vi "Program_EBN_Yann_Berton.vi"() -> ()   [LabVIEW 2020]
uses:
  <instrlib>/Keithley 27XX/Public/Configure/Measurement Specific/Configure Thermocouple.vi
  <instrlib>/Keithley 27XX/Public/Configure/Measurement Specific/Configure FRTD.vi
  <instrlib>/Keithley 27XX/Keithley 27XX.lvlib
panel:
  in  "Number of samples allowed":dbl=15.0
  out "Close 50 mbar valve":bool
  out "T_ts_in_mid (wall)":dbl
  out "T_ts_in_top (wall)":dbl
  out "T_out_ts_mid (wall)":dbl
  out "T_out_ts_bot (wall)":dbl
  out "Counter":dbl
  out "T_PH_surf4":dbl
  out "T_PH_surf3":dbl
  out "TCHF_bot":dbl
  out "TCHF_top":dbl
  out "T3_bot":dbl
  out "T3_mid":dbl
  out "T3_top":dbl
  out "T2_top":dbl
  out "T2_mid":dbl
  out "T2_bot":dbl
  out "T1_top":dbl
  out "T1_mid":dbl
  out "T1_bot":dbl
  out "T_PH_surf2":dbl
  out "Absolute pressure":dynamicdata(graph)
  out "Pressure drop":dynamicdata(graph)
  out "Temperatures":dynamicdata(graph)
  in  "Porta RS232 Keithley 2701":refnum<visa-resource-name>="COM1"
  in  "Aquisition {Sample/s]":u32=1
  in  "stop":bool
  out "stop flag":bool
  out "V_TS_corr2":dbl
  out "P_reservoir (kPa)":dbl
  out "P_TS_in (kPa)":dbl
  out "P_pump_in (kPa)":dbl
  out "mass (kg/s)":dbl
  out "0-50 mbar (kPa)":dbl
  out "0-2 bar (kPa)":dbl
  out "T_ph_in (imm)":dbl
  out "T_amb":dbl
  out "T_reserv_bot":dbl
  out "T_reser_top":dbl
  out "T_TS_out_top (wall)":dbl
  out "T_TS_out (imm)":dbl
  out "T_PH_surf1":dbl
  out "T_PH_in (wall)":dbl
  out "T_TS_in (imm)":dbl
  out "T_TS_in_bot (wall)":dbl
  out "T_pump_in":dbl
  in  "File":path=path "C:/test.lvm" caption="Filename"
  in  "Save":bool caption="Enable"
  out "0-5 bar (kPa)":dbl
  out "Tcj ch201":dbl
  # "SAVING DATA"
  # "Pre-heater temperatures"
  # "Test section temperatures"
  # "85 mm mm"
  # "40 mm"
  # "62.5 mm mm"
  # "665 mm"
  # "1347 mm mm"
  # "115 mm mm"
  # "809 mm"
  # "1585 mm mm"
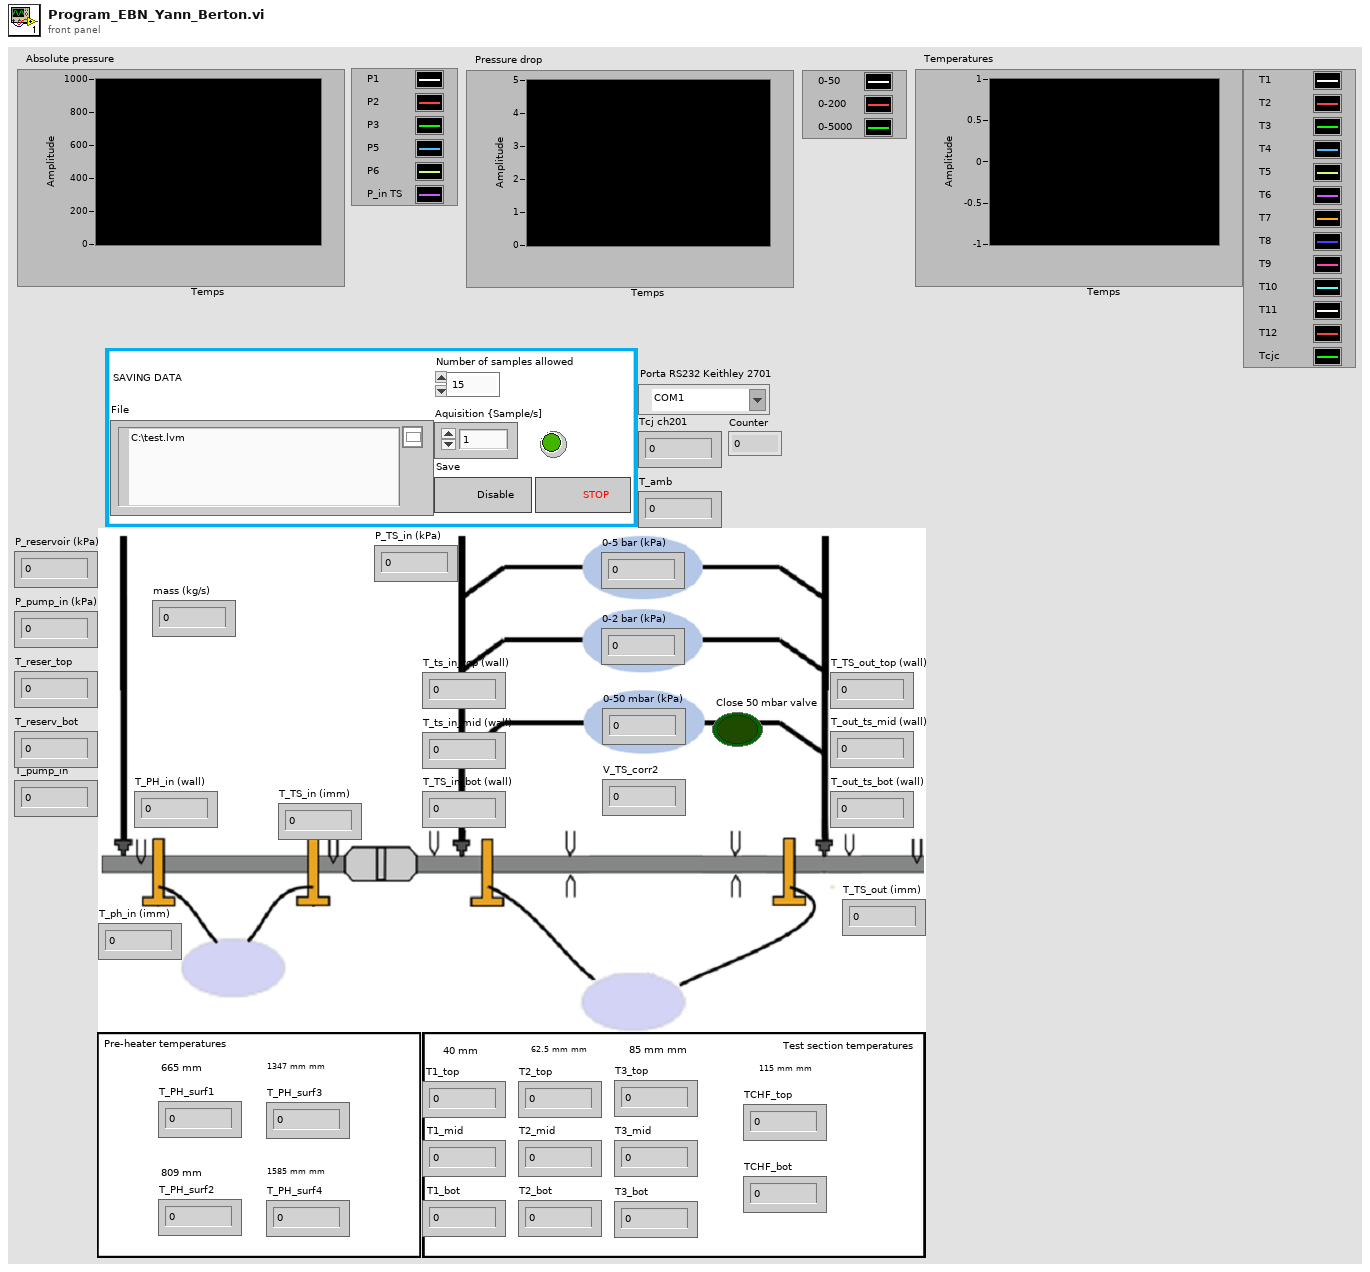
[diagram p1: front panel]
types:
  T1 = cluster{"Baud Rate (9600)":u32, "Flow Control (1: XON/XOFF)":u16, "Termination Char (0:CR)":u16}
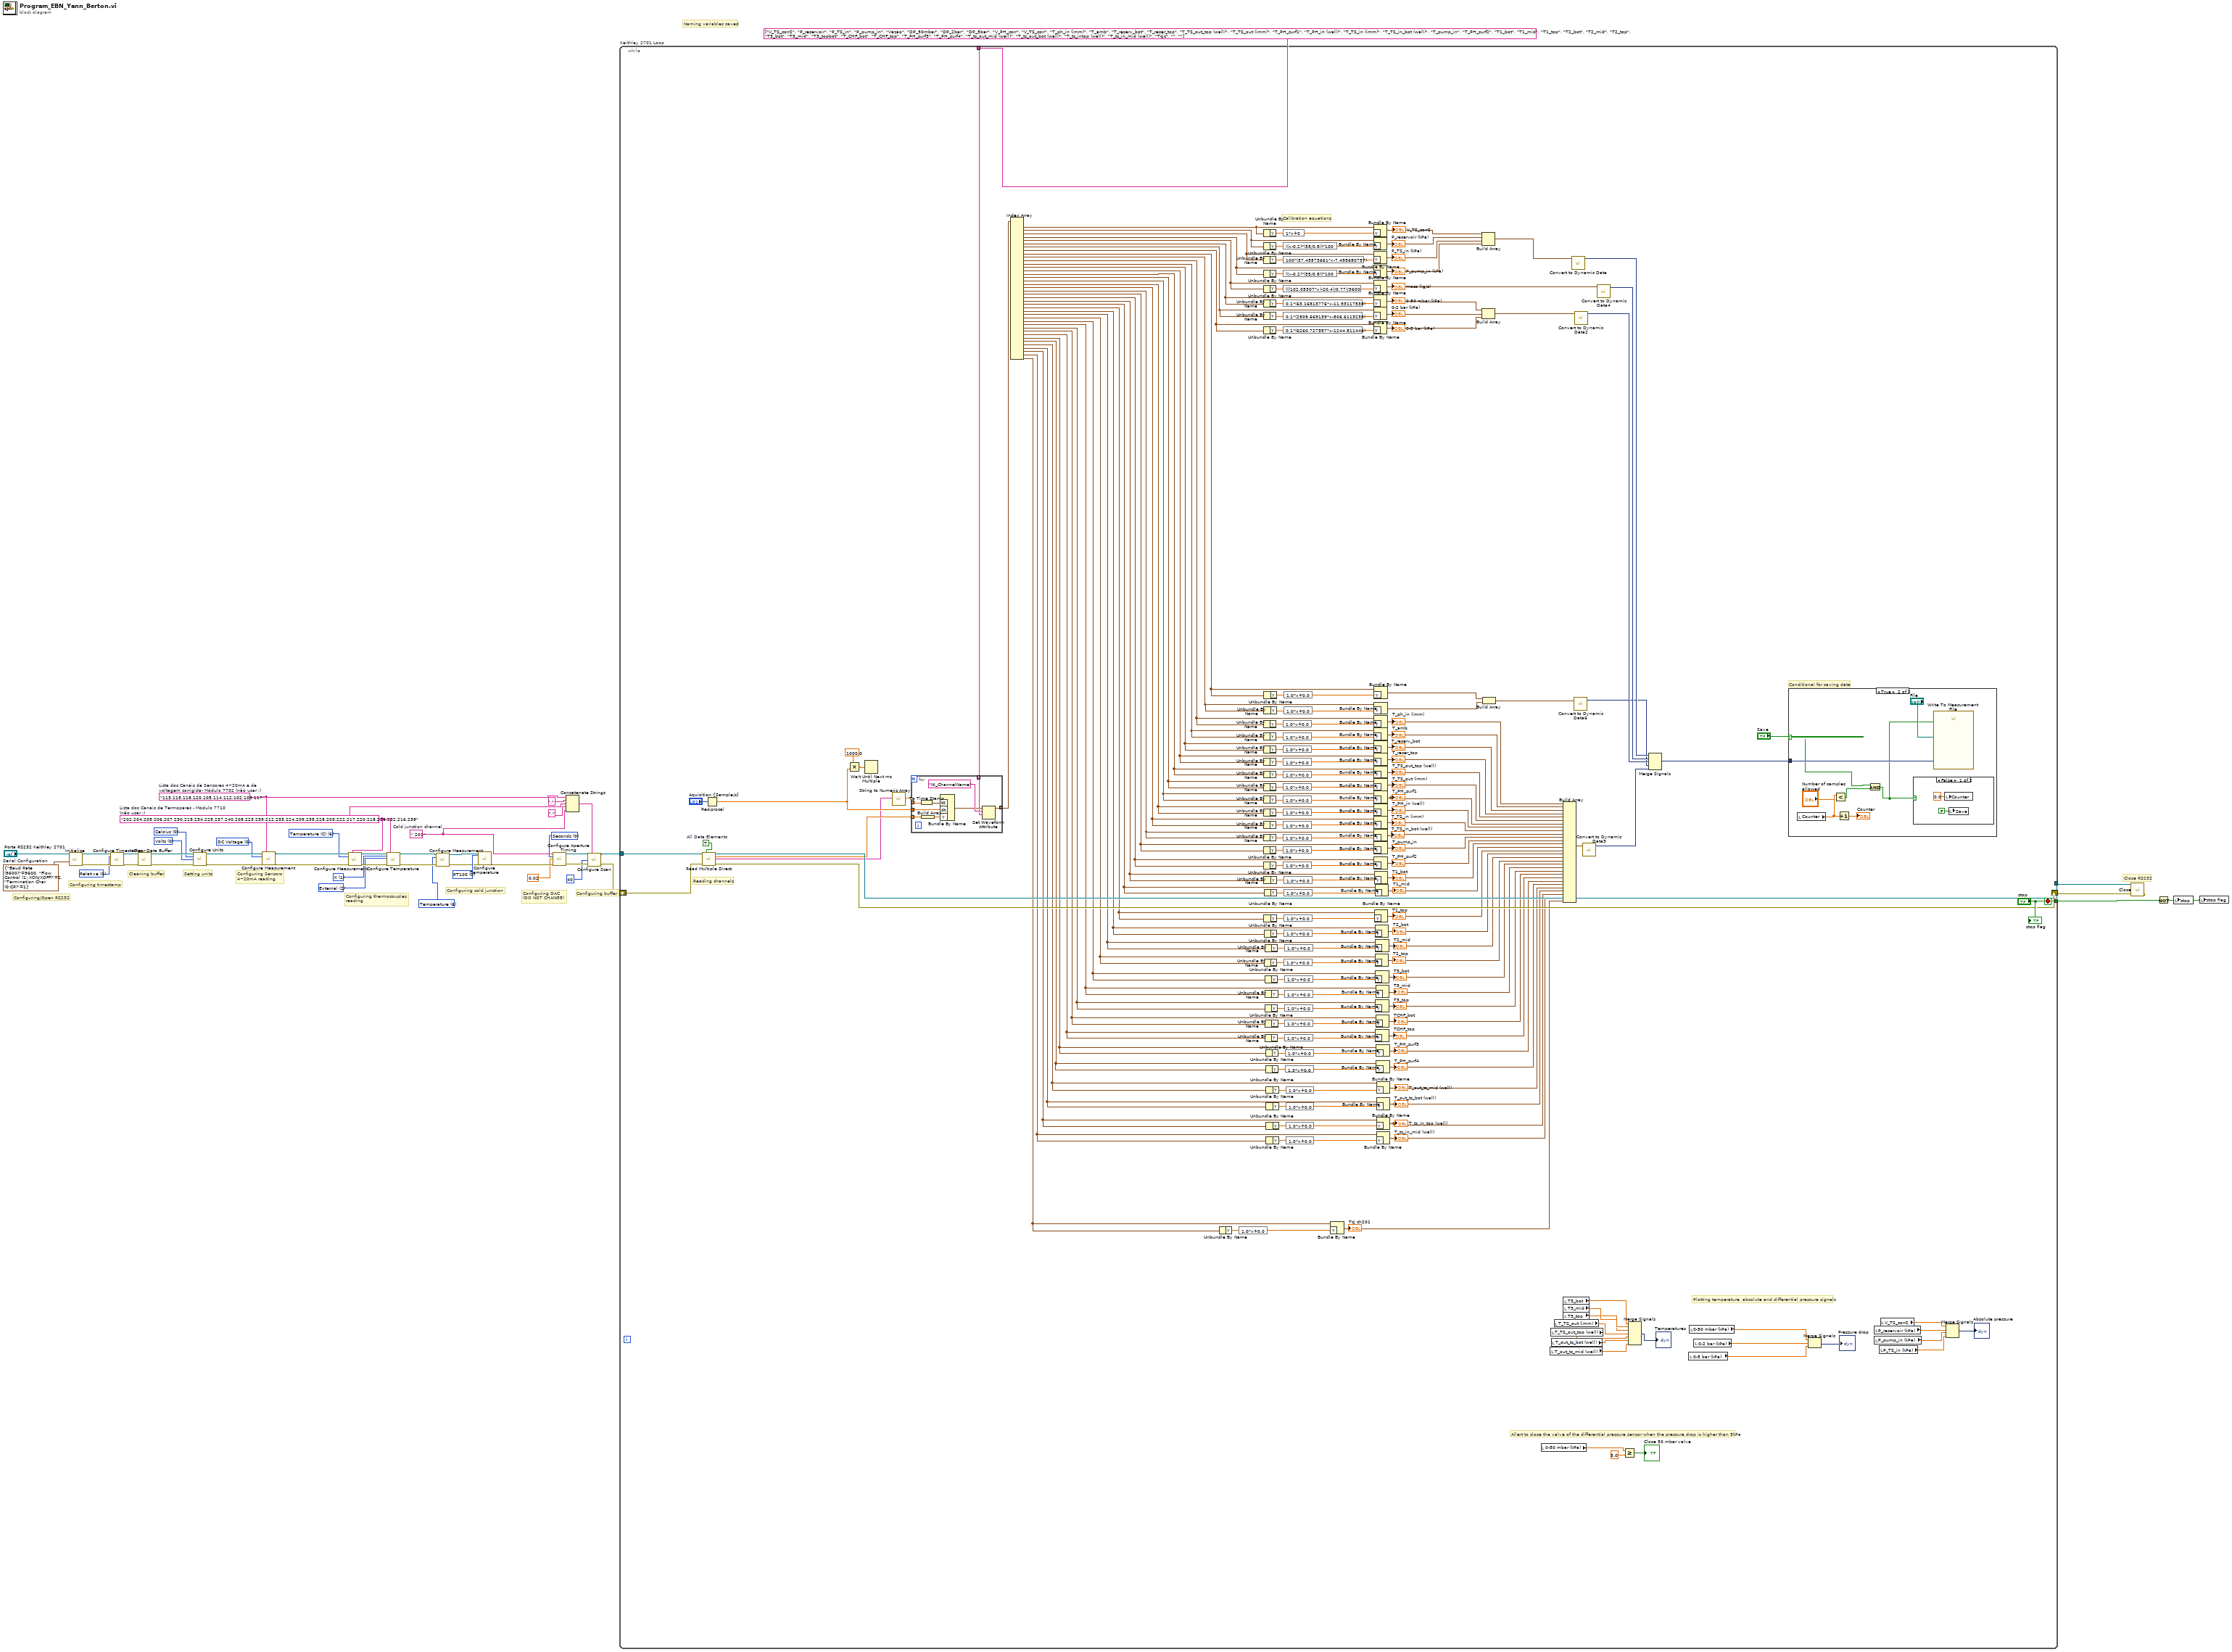
[diagram p0: block diagram]
diagram:
  w15 = u16 0 items=["PT100", "D100", "F100", "PT3916", "PT385", "USER"] ("FRTD Type (0: PT100)")
  w17 = u16 6 items=["DC Voltage", "AC Voltage", "DC Current", "AC Current", "Resistance", "Four-Wire Resistance", "Temperature", "Frequency", "Period", "Continuity"] ("Function (0: DC Voltage)")
  w1 = " 201"  # Cold junction channel
  w23 = "202,204,205,206,207,230,219,234,225,237,240,208,223,239,212,233,224,209,235,228,203,222,217,220,218,226,232,216,238"  # Lista dos Canais de Termopares - Módulo 7710 (não usar :)
  w31 = "113,115,118,120,105,114,112,102,109,117"  # Lista dos Canais de Sensores 4~20mA e de voltagem corrigida- Módulo 7702 (não usar :)
  w12 = u16 0 items=["Seconds", "Power Line Cycles"] ("Timing Units (0: Seconds)")
  w20 = u16 2 items=["Simulated", "Internal", "External"] ("Reference Junction Type (0: Simulated)")
  w21 = u16 1 items=["J", "K", "T", "E", "R", "S", "B", "N"] ("Thermocouple Type (1: K)")
  w32 = u16 0 items=["Volts", "dB"] ("DC Voltage (0: V)")
  w33 = u16 0 items=["Celsius", "Fahrenheit", "Kelvin"] ("Temperature (0: Celsius)")
  w25 = u16 6 items=["DC Voltage", "AC Voltage", "DC Current", "AC Current", "Resistance", "Four-Wire Resistance", "Temperature (C)", "Frequency", "Period", "Continuity"] ("Function (0: DC Voltage)")
  w28 = u16 0 items=["DC Voltage", "AC Voltage", "DC Current", "AC Current", "Resistance", "Four-Wire Resistance", "Temperature (C)", "Frequency", "Period", "Continuity"] ("Function (0: DC Voltage)")
  w41 = T1 {"Baud Rate (9600)"=9600, "Flow Control (1: XON/XOFF)"=2, "Termination Char (0:CR)"=1}  # Serial Configuration
  w38 = u16 0 items=["Relative", "Real Time Clock"] ("Timestamp Type (0: Relative)")
  # "Configuring cold junction"
  # "Naming variables saved"
  # "Close RS232"
  # "Configuring buffer"
  # "Configuring DAC \n(DO NOT CHANGE)"
  # "Configuring thermocouples\nreading"
  # "Configuring Sensors \n4~20mA reading"
  # "Setting units"
  # "Cleaning buffer"
  # "Configuring timestamp"
  # "Configuring/Open RS232"
  n1 = call <instrlib>:"Initialize.vi"("VISA resource name"="Porta RS232 Keithley 2701", "Serial Configuration"=w41) -> ("VISA resource name out"=w40:refnum<visa-resource-name>, "error out"=w39:errorcluster)  [unwired: 12 in]
  n2 = call <instrlib>:"Configure Timestamp.vi"("VISA resource name"=w40, "Timestamp Type (0: Relative)"=w38, "error in (no error)"=w39) -> ("VISA resource name out"=w37:refnum<visa-resource-name>, "error out"=w36:errorcluster)  [unwired: 11 in]
  n3 = call <instrlib>:"Clear Data Buffer.vi"("VISA resource name"=w37, "error in (no error)"=w36) -> ("VISA resource name out"=w35:refnum<visa-resource-name>, "error out"=w34:errorcluster)  [unwired: 12 in]
  n4 = call <instrlib>:"Configure Units.vi"("VISA resource name"=w35, "Temperature (0: Celsius)"=w33, "DC Voltage (0: V)"=w32, "error in (no error)"=w34) -> ("VISA resource name out"=w29:refnum<visa-resource-name>, "error out"=w30:errorcluster)  [unwired: 10 in]
  n5 = call <instrlib>:"Configure Measurement.vi"("VISA resource name"=w29, "Scan List (Empty)"=w31, "Function (0: DC Voltage)"=w28, "error in (no error)"=w30) -> ("VISA resource name out"=w27:refnum<visa-resource-name>, "error out"=w26:errorcluster)  [unwired: 10 in]
  n6 = call <instrlib>:"Configure Measurement.vi"("VISA resource name"=w27, "Scan List (Empty)"=w23, "Function (0: DC Voltage)"=w25, "error in (no error)"=w26) -> ("VISA resource name out"=w24:refnum<visa-resource-name>, "error out"=w22:errorcluster)  [unwired: 10 in]
  n7 = call-poly <instrlib>:"Configure Temperature.vi"("VISA resource name"=w24, "Thermocouple Type (1: K)"=w21, "Reference Junction Type (0: Simulated)"=w20, "error in (no error)"=w22, "Scan List (Empty)"=w23) -> ("VISA resource name out"=w19:refnum<visa-resource-name>, "error out"=w18:errorcluster)  [unwired: 13 in]
  n8 = call <instrlib>:"Configure Measurement.vi"("VISA resource name"=w19, "Function (0: DC Voltage)"=w17, "error in (no error)"=w18) -> ("VISA resource name out"=w16:refnum<visa-resource-name>, "error out"=w14:errorcluster)  [unwired: 11 in]
  n9 = call-poly <instrlib>:"Configure Temperature.vi"("VISA resource name"=w16, "FRTD Type (0: PT100)"=w15, "error in (no error)"=w14) -> ("error out"=w13:errorcluster)  [unwired: 15 in, 1 out]
  n10 = call <instrlib>:"Configure Aperture Timing.vi"("VISA resource name"=w1, "Timing Units (0: Seconds)"=w12, "Timing Value (0.020)"=0.02, "error in (no error)"=w13) -> ("VISA resource name out"=w9:refnum<visa-resource-name>, "error out"=w8:errorcluster)  [unwired: 10 in]
  n11 = Concatenate Strings(w31, "," ("string"), w23, "," ("string"), w1) -> (w10:string)
  n12 = call <instrlib>:"Configure Scan.vi"("VISA resource name"=w9, "Channel List (101:110)"=w10, "Sample Count (100)"=40 ("Sample Count (10)"), "error in (no error)"=w8) -> ("VISA resource name out"=w6:refnum<visa-resource-name>, "error out"=w7:errorcluster)  [unwired: 10 in]
  n13 = while "Keithley 2701 Loop" {
    tunnel: w6 -> [w197]
    tunnel: [w194] -> w4
    shift-right: [w195] -> w3
    shift-left: w7 -> [w196]
    tunnel: string[] ["V_TS_corr2", "P_reservoir", "P_TS_in", "P_pump_in", "Vazao", "DP_50mbar", "DP_2bar", "DP_5bar", "V_PH_corr", "V_TS_corr", "T_ph_in (imm)", "T_amb", "T_reserv_bot", "T_reser_top", "T_TS_out_top (wall)", "T_TS_out (imm)", "T_PH_surf1", "T_PH_in (wall)", "T_TS_in (imm)", "T_TS_in_bot (wall)", "T_pump_in", "T_PH_surf2", "T1_bot", "T1_mid", "T1_top", "T2_bot", "T2_mid", "T2_top", "T3_bot", "T3_mid", "T3_topbot", "T_CHF_bot", "T_CHF_top", "T_PH_surf3", "T_PH_surf4", "T_ts_out_mid (wall)", "T_ts_out_bot (wall)", "T_ts_intop (wall)", "T_ts_in_mid (wall)", "Tcjc", "", ""] -> [w248]
    tunnel: ["stop"] -> w2
    stop <- "stop" stop-if-true
    w190 = TRUE  # All Data Elements
    # "Allert to close the valve of the differential pressure sensor when the pressure drop is higher than 5kPa"
    # "Plotting temperature, absolute and differential pressure signals"
    # "Conditional for saving data"
    # "Calibration equations"
    # "Reading channels"
    n14 = call <instrlib>:"Read Multiple Direct.vi"("VISA resource name"=w197, "All Data Elements (False)"=w190, "error in (no error)"=w196) -> ("VISA resource name out"=w194:refnum<visa-resource-name>, "Measurement Data"=w193:dbl[], "Time Stamp"=w192:string[], "error out"=w195:errorcluster)  [unwired: 7 in, 2 out]
    n15 = Reciprocal(x="Aquisition {Sample/s]") -> (1/x=w249:dbl)
    n16 = Multiply(x=1000.0 ("y"), y=w249) -> (x*y=w250:dbl)
    n17 = Wait Until Next ms Multiple(millisecond multiple=w250) -> ()  [unwired: 1 out]
    n18 = call <instrlib>:"String to Numeric Array.vi"("String Array"=w192) -> ("Numeric Array"=w191:dbl[])  [unwired: 10 in]
    n19 = for {
      tunnel: w191 -> [w271] mode=indexing
      tunnel: w193 -> [w269] mode=indexing
      tunnel: w249 -> [w267]
      tunnel: w248 -> [w264] mode=indexing
      tunnel: [w263] -> w247 mode=indexing
      n20 = To Time Stamp(1:w271) -> (0:w270:timestamp)
      n21 = Build Array(w269) -> (w268:dbl[])
      n22 = Bundle By Name("t0"=w270, "dt"=w267, "Y"=w268) -> (w265:waveform(dbl))  [unwired: 1 in]
      n23 = Set Waveform Attribute(5:w264, 6:"NI_ChannelName" ("name"), 7:w265) -> (3:w263:waveform(dbl))  [unwired: 1 in, 2 out]
    }
    n24 = Index Array(array=w247) -> (element #1=w161:waveform(dbl), element #2=w160:waveform(dbl), element #3=w159:waveform(dbl), element #4=w158:waveform(dbl), element #5=w157:waveform(dbl), element #6=w156:waveform(dbl), element #7=w54:waveform(dbl), element #8=w155:waveform(dbl), element #9=w148:waveform(dbl), element #10=w145:waveform(dbl), element #11=w202:waveform(dbl), element #12=w203:waveform(dbl), element #13=w204:waveform(dbl), element #14=w205:waveform(dbl), element #15=w206:waveform(dbl), element #16=w207:waveform(dbl), element #17=w208:waveform(dbl), element #18=w209:waveform(dbl), element #19=w210:waveform(dbl), element #20=w211:waveform(dbl), element #21=w212:waveform(dbl), element #22=w139:waveform(dbl), element #23=w136:waveform(dbl), element #24=w131:waveform(dbl), element #25=w130:waveform(dbl), element #26=w123:waveform(dbl), element #27=w122:waveform(dbl), element #28=w121:waveform(dbl), element #29=w114:waveform(dbl), element #30=w113:waveform(dbl), element #31=w112:waveform(dbl), element #32=w107:waveform(dbl), element #33=w106:waveform(dbl), element #34=w78:waveform(dbl), element #35=w77:waveform(dbl), element #36=w70:waveform(dbl), element #37=w69:waveform(dbl), element #38=w64:waveform(dbl), element #39=w60:waveform(dbl), element #40=w52:waveform(dbl))  [unwired: 40 in]
    n25 = Unbundle By Name(w52) -> ("Y"=w201:dbl[])
    n26 = expression code="1.0*x+0.0"(w201) -> (w176:dbl[])
    n27 = Unbundle By Name(w161) -> ("Y"=w245:dbl[])
    n28 = Unbundle By Name(w160) -> ("Y"=w242:dbl[])
    n29 = Unbundle By Name(w159) -> ("Y"=w244:dbl[])
    n30 = Unbundle By Name(w158) -> ("Y"=w237:dbl[])
    n31 = Unbundle By Name(w157) -> ("Y"=w241:dbl[])
    n32 = Unbundle By Name(w156) -> ("Y"=w238:dbl[])
    n33 = Unbundle By Name(w54) -> ("Y"=w235:dbl[])
    n34 = Unbundle By Name(w155) -> ("Y"=w214:dbl[])
    n35 = Unbundle By Name(w202) -> ("Y"=w233:dbl[])
    n36 = Unbundle By Name(w203) -> ("Y"=w231:dbl[])
    n37 = Unbundle By Name(w204) -> ("Y"=w232:dbl[])
    n38 = Unbundle By Name(w205) -> ("Y"=w227:dbl[])
    n39 = Unbundle By Name(w206) -> ("Y"=w228:dbl[])
    n40 = Unbundle By Name(w207) -> ("Y"=w230:dbl[])
    n41 = Unbundle By Name(w208) -> ("Y"=w229:dbl[])
    n42 = Unbundle By Name(w209) -> ("Y"=w223:dbl[])
    n43 = Unbundle By Name(w210) -> ("Y"=w226:dbl[])
    n44 = Unbundle By Name(w211) -> ("Y"=w225:dbl[])
    n45 = Unbundle By Name(w212) -> ("Y"=w224:dbl[])
    n46 = Unbundle By Name(w139) -> ("Y"=w141:dbl[])
    n47 = Unbundle By Name(w148) -> ("Y"=w150:dbl[])
    n48 = Unbundle By Name(w145) -> ("Y"=w146:dbl[])
    n49 = Unbundle By Name(w136) -> ("Y"=w137:dbl[])
    n50 = Unbundle By Name(w130) -> ("Y"=w132:dbl[])
    n51 = Unbundle By Name(w131) -> ("Y"=w135:dbl[])
    n52 = Unbundle By Name(w123) -> ("Y"=w129:dbl[])
    n53 = Unbundle By Name(w121) -> ("Y"=w125:dbl[])
    n54 = Unbundle By Name(w122) -> ("Y"=w127:dbl[])
    n55 = Unbundle By Name(w114) -> ("Y"=w115:dbl[])
    n56 = Unbundle By Name(w112) -> ("Y"=w119:dbl[])
    n57 = Unbundle By Name(w106) -> ("Y"=w109:dbl[])
    n58 = Unbundle By Name(w113) -> ("Y"=w117:dbl[])
    n59 = Unbundle By Name(w107) -> ("Y"=w111:dbl[])
    n60 = Unbundle By Name(w78) -> ("Y"=w82:dbl[])
    n61 = Unbundle By Name(w77) -> ("Y"=w80:dbl[])
    n62 = Unbundle By Name(w70) -> ("Y"=w71:dbl[])
    n63 = Unbundle By Name(w69) -> ("Y"=w73:dbl[])
    n64 = Unbundle By Name(w64) -> ("Y"=w66:dbl[])
    n65 = Unbundle By Name(w60) -> ("Y"=w61:dbl[])
    n66 = expression code="1*x+0"(w245) -> (w246:dbl[])
    n67 = expression code="((x-0.2)*(35/0.8))*100"(w242) -> (w243:dbl[])
    n68 = expression code="100*(37.49573661*x-7.495680797)"(w244) -> (w200:dbl[])
    n69 = expression code="((x-0.2)*(35/0.8))*100"(w237) -> (w236:dbl[])
    n70 = expression code="(((102.05307*x)-20.4)/0.77)/3600"(w241) -> (w240:dbl[])
    n71 = expression code="0.1*(63.16813776*x-11.93117538)"(w238) -> (w239:dbl[])
    n72 = expression code="0.1*(2509.669139*x-506.6113235)"(w235) -> (w234:dbl[])
    n73 = expression code="0.1*(6260.727357*x-1244.811446)"(w214) -> (w215:dbl[])
    n74 = expression code="1.0*x+0.0"(w233) -> (w177:dbl[])
    n75 = expression code="1.0*x+0.0"(w231) -> (w178:dbl[])
    n76 = expression code="1.0*x+0.0"(w232) -> (w188:dbl[])
    n77 = expression code="1.0*x+0.0"(w227) -> (w187:dbl[])
    n78 = expression code="1.0*x+0.0"(w228) -> (w186:dbl[])
    n79 = expression code="1.0*x+0.0"(w230) -> (w185:dbl[])
    n80 = expression code="1.0*x+0.0"(w229) -> (w184:dbl[])
    n81 = expression code="1.0*x+0.0"(w223) -> (w183:dbl[])
    n82 = expression code="1.0*x+0.0"(w226) -> (w182:dbl[])
    n83 = expression code="1.0*x+0.0"(w225) -> (w181:dbl[])
    n84 = expression code="1.0*x+0.0"(w224) -> (w180:dbl[])
    n85 = expression code="1.0*x+0.0"(w141) -> (w140:dbl[])
    n86 = expression code="1.0*x+0.0"(w150) -> (w149:dbl[])
    n87 = expression code="1.0*x+0.0"(w146) -> (w147:dbl[])
    n88 = expression code="1.0*x+0.0"(w137) -> (w138:dbl[])
    n89 = expression code="1.0*x+0.0"(w132) -> (w133:dbl[])
    n90 = expression code="1.0*x+0.0"(w135) -> (w134:dbl[])
    n91 = expression code="1.0*x+0.0"(w129) -> (w128:dbl[])
    n92 = expression code="1.0*x+0.0"(w125) -> (w124:dbl[])
    n93 = expression code="1.0*x+0.0"(w127) -> (w126:dbl[])
    n94 = expression code="1.0*x+0.0"(w115) -> (w116:dbl[])
    n95 = expression code="1.0*x+0.0"(w119) -> (w120:dbl[])
    n96 = expression code="1.0*x+0.0"(w109) -> (w108:dbl[])
    n97 = expression code="1.0*x+0.0"(w117) -> (w118:dbl[])
    n98 = expression code="1.0*x+0.0"(w111) -> (w110:dbl[])
    n99 = expression code="1.0*x+0.0"(w82) -> (w81:dbl[])
    n100 = expression code="1.0*x+0.0"(w80) -> (w79:dbl[])
    n101 = expression code="1.0*x+0.0"(w71) -> (w72:dbl[])
    n102 = expression code="1.0*x+0.0"(w73) -> (w74:dbl[])
    n103 = expression code="1.0*x+0.0"(w66) -> (w65:dbl[])
    n104 = expression code="1.0*x+0.0"(w61) -> (w62:dbl[])
    n105 = Bundle By Name(cluster=w52, "Y"=w176) -> (w53:waveform(dbl))
    "Tcj ch201" <- w53
    n106 = Bundle By Name(cluster=w161, "Y"=w246) -> (w165:waveform(dbl))
    "V_TS_corr2" <- w165
    n107 = Bundle By Name(cluster=w160, "Y"=w243) -> (w164:waveform(dbl))
    "P_reservoir (kPa)" <- w164
    n108 = Bundle By Name(cluster=w159, "Y"=w200) -> (w163:waveform(dbl))
    "P_TS_in (kPa)" <- w163
    n109 = Bundle By Name(cluster=w158, "Y"=w236) -> (w162:waveform(dbl))
    "P_pump_in (kPa)" <- w162
    n110 = Bundle By Name(cluster=w157, "Y"=w240) -> (w199:waveform(dbl))
    "mass (kg/s)" <- w199
    n111 = Bundle By Name(cluster=w156, "Y"=w239) -> (w56:waveform(dbl))
    "0-50 mbar (kPa)" <- w56
    n112 = Bundle By Name(cluster=w54, "Y"=w234) -> (w218:waveform(dbl))
    "0-2 bar (kPa)" <- w218
    n113 = Bundle By Name(cluster=w155, "Y"=w215) -> (w213:waveform(dbl))
    "0-5 bar (kPa)" <- w213
    n114 = Bundle By Name(cluster=w148, "Y"=w149) -> (w143:waveform(dbl))
    n115 = Bundle By Name(cluster=w145, "Y"=w147) -> (w142:waveform(dbl))
    n116 = Bundle By Name(cluster=w202, "Y"=w177) -> (w105:waveform(dbl))
    "T_ph_in (imm)" <- w105
    n117 = Bundle By Name(cluster=w203, "Y"=w178) -> (w104:waveform(dbl))
    "T_amb" <- w104
    n118 = Bundle By Name(cluster=w204, "Y"=w188) -> (w103:waveform(dbl))
    "T_reserv_bot" <- w103
    n119 = Bundle By Name(cluster=w205, "Y"=w187) -> (w102:waveform(dbl))
    "T_reser_top" <- w102
    n120 = Bundle By Name(cluster=w206, "Y"=w186) -> (w101:waveform(dbl))
    "T_TS_out_top (wall)" <- w101
    n121 = Bundle By Name(cluster=w207, "Y"=w185) -> (w100:waveform(dbl))
    "T_TS_out (imm)" <- w100
    n122 = Bundle By Name(cluster=w208, "Y"=w184) -> (w99:waveform(dbl))
    "T_PH_surf1" <- w99
    n123 = Bundle By Name(cluster=w209, "Y"=w183) -> (w98:waveform(dbl))
    "T_PH_in (wall)" <- w98
    n124 = Bundle By Name(cluster=w210, "Y"=w182) -> (w97:waveform(dbl))
    "T_TS_in (imm)" <- w97
    n125 = Bundle By Name(cluster=w211, "Y"=w181) -> (w96:waveform(dbl))
    "T_TS_in_bot (wall)" <- w96
    n126 = Bundle By Name(cluster=w212, "Y"=w180) -> (w95:waveform(dbl))
    "T_pump_in" <- w95
    n127 = Bundle By Name(cluster=w139, "Y"=w140) -> (w94:waveform(dbl))
    "T_PH_surf2" <- w94
    n128 = Bundle By Name(cluster=w136, "Y"=w138) -> (w93:waveform(dbl))
    "T1_bot" <- w93
    n129 = Bundle By Name(cluster=w130, "Y"=w133) -> (w91:waveform(dbl))
    "T1_top" <- w91
    n130 = Bundle By Name(cluster=w131, "Y"=w134) -> (w92:waveform(dbl))
    "T1_mid" <- w92
    n131 = Bundle By Name(cluster=w123, "Y"=w128) -> (w90:waveform(dbl))
    "T2_bot" <- w90
    n132 = Bundle By Name(cluster=w121, "Y"=w124) -> (w88:waveform(dbl))
    "T2_top" <- w88
    n133 = Bundle By Name(cluster=w122, "Y"=w126) -> (w89:waveform(dbl))
    "T2_mid" <- w89
    n134 = Bundle By Name(cluster=w114, "Y"=w116) -> (w87:waveform(dbl))
    "T3_bot" <- w87
    n135 = Bundle By Name(cluster=w112, "Y"=w120) -> (w85:waveform(dbl))
    "T3_top" <- w85
    n136 = Bundle By Name(cluster=w106, "Y"=w108) -> (w83:waveform(dbl))
    "TCHF_top" <- w83
    n137 = Bundle By Name(cluster=w113, "Y"=w118) -> (w86:waveform(dbl))
    "T3_mid" <- w86
    n138 = Bundle By Name(cluster=w107, "Y"=w110) -> (w84:waveform(dbl))
    "TCHF_bot" <- w84
    n139 = Bundle By Name(cluster=w78, "Y"=w81) -> (w76:waveform(dbl))
    "T_PH_surf3" <- w76
    n140 = Bundle By Name(cluster=w77, "Y"=w79) -> (w75:waveform(dbl))
    "T_PH_surf4" <- w75
    n141 = Bundle By Name(cluster=w70, "Y"=w72) -> (w68:waveform(dbl))
    "T_out_ts_mid (wall)" <- w68
    n142 = Bundle By Name(cluster=w69, "Y"=w74) -> (w67:waveform(dbl))
    "T_out_ts_bot (wall)" <- w67
    n143 = Bundle By Name(cluster=w64, "Y"=w65) -> (w63:waveform(dbl))
    "T_ts_in_top (wall)" <- w63
    n144 = Bundle By Name(cluster=w60, "Y"=w62) -> (w59:waveform(dbl))
    "T_ts_in_mid (wall)" <- w59
    n145 = Build Array(w165, w164, w163, w162) -> (w189:waveform(dbl)[])
    n146 = Build Array(w56, w218, w213) -> (w222:waveform(dbl)[])
    n147 = Build Array(w143, w142) -> (w144:waveform(dbl)[])
    n148 = local read "0-50 mbar (kPa)"() -> (w55:dbl)
    n149 = local read "T_out_ts_mid (wall)"() -> (w47:dbl)
    n150 = local read "T_TS_out_top (wall)"() -> (w49:dbl)
    n151 = local read "T_out_ts_bot (wall)"() -> (w48:dbl)
    n152 = local read "T_TS_out (imm)"() -> (w171:dbl)
    n153 = Build Array(w105, w104, w103, w102, w101, w100, w99, w98, w97, w96, w95, w94, w93, w92, w91, w90, w89, w88, w87, w86, w85, w84, w83, w76, w75, w68, w67, w63, w59, w53) -> (w179:waveform(dbl)[])
    n154 = local read "T3_bot"() -> (w174:dbl)
    n155 = local read "T3_mid"() -> (w173:dbl)
    n156 = local read "T3_top"() -> (w172:dbl)
    n157 = call "Convert to Dynamic Data"("Array of Waveforms"=w189) -> ("Dynamic Data Type"=w219:dynamicdata)  [unwired: 3 in]
    n158 = call "Convert to Dynamic Data6"("Array of Waveforms"=w144) -> ("Dynamic Data Type"=w50:dynamicdata)  [unwired: 3 in]
    n159 = call "Convert to Dynamic Data2"("Array of Waveforms"=w222) -> ("Dynamic Data Type"=w220:dynamicdata)  [unwired: 3 in]
    n160 = call "Convert to Dynamic Data3"("Array of Waveforms"=w179) -> ("Dynamic Data Type"=w51:dynamicdata)  [unwired: 3 in]
    n161 = call "Convert to Dynamic Data4"("Waveform"=w199) -> ("Dynamic Data Type"=w198:dynamicdata)  [unwired: 3 in]
    n162 = Greater Or Equal?(x=w55, y=5.0) -> (x >= y?=→"Close 50 mbar valve":bool)
    n163 = Merge Signals(w174, w173, w172, w171, w49, w48, w47) -> (→"Temperatures":dynamicdata)
    n164 = Merge Signals(w219, w198, w220, w50, w51) -> (w221:dynamicdata)
    n165 = local read "0-5 bar (kPa)"() -> (w166:dbl)
    n166 = local read "0-50 mbar (kPa)"() -> (w168:dbl)
    n167 = local read "0-2 bar (kPa)"() -> (w167:dbl)
    n168 = case shown="True" "Save" {
      selector: "Save" -> [_ w256]
      tunnel: w221 -> [_ w260]
      frame False {
      }
      frame True {
        n169 = local read "Counter"() -> (w257:dbl)
        n170 = Less?(x=w257, y="Number of samples allowed") -> (x < y?=w255:bool)
        n171 = Increment(x=w257) -> (x+1=→"Counter":dbl)
        n172 = And(x=w256, y=w255) -> (x .and. y?=w254:bool)
        n173 = case shown="False" w254 {
          frame False {
            n174 = local write "Counter"(0.0 ("Counter")) -> ()
            n175 = local write "Save"(FALSE ("Save")) -> ()
          }
          frame True {
          }
        }
        n176 = call "Write To Measurement File"("Signals"=w260, "Enable"=w254, "Filename"="File") -> ()  [unwired: 14 in, 3 out]
      }
    }
    n177 = Merge Signals(w168, w167, w166) -> (→"Pressure drop":dynamicdata)
    n178 = local read "P_reservoir (kPa)"() -> (w153:dbl)
    n179 = local read "P_pump_in (kPa)"() -> (w152:dbl)
    n180 = local read "P_TS_in (kPa)"() -> (w151:dbl)
    n181 = local read "V_TS_corr2"() -> (w154:dbl)
    n182 = Merge Signals(w154, w153, w152, w151) -> (→"Absolute pressure":dynamicdata)
    "stop flag" <- "stop"
  }
  n183 = call <instrlib>:"Close.vi"("VISA resource name"=w4, "error in (no error)"=w3) -> ()  [unwired: 13 in, 1 out]
  n184 = Not(x=w2) -> (.not. x?=w44:bool)
  n185 = local write "stop"(w44) -> ()
  n186 = local write "stop flag"(w44) -> ()
